vi "read_params.vi"(8 "error in (no error)":errorcluster, 11 "OrthogonalMatchingPursuit in":refnum<class "OrthogonalMatchingPursuit.lvclass">) -> (0 "error out":errorcluster, 2 "params":T1={"n_nonzero_coefs"={"n_nonzero_coefs_type"="None", "n_nonzero_coefs_int"=0.0}, "tol"={"tol_type"="None", "tol_float"=0.0}, "fit_intercept"=TRUE, "normalize"=TRUE, "precompute"={"precompute_type"="auto", "precompute_bool"=FALSE}}, 3 "OrthogonalMatchingPursuit out":refnum<class "OrthogonalMatchingPursuit.lvclass">)   [LabVIEW 2020, in "OrthogonalMatchingPursuit.lvclass"]
uses:
  OrthogonalMatchingPursuit.lvclass
  Controls/orthogonal_matching_pursuit_params.ctl
  OrthogonalMatchingPursuit.lvclass/OrthogonalMatchingPursuit.ctl
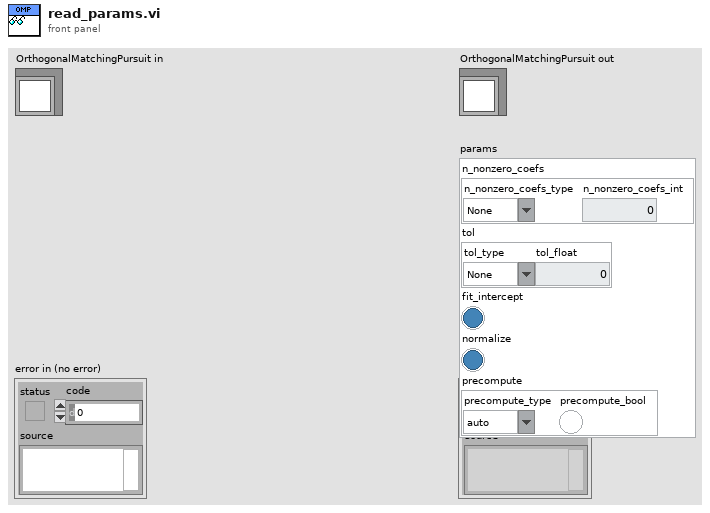
[diagram p1: front panel]
types:
  T1 = typedef "orthogonal_matching_pursuit_params.ctl" = cluster{"n_nonzero_coefs":cluster{"n_nonzero_coefs_type":string, "n_nonzero_coefs_int":dbl}, "tol":cluster{"tol_type":string, "tol_float":dbl}, "fit_intercept":bool, "normalize":bool, "precompute":cluster{"precompute_type":string, "precompute_bool":bool}}
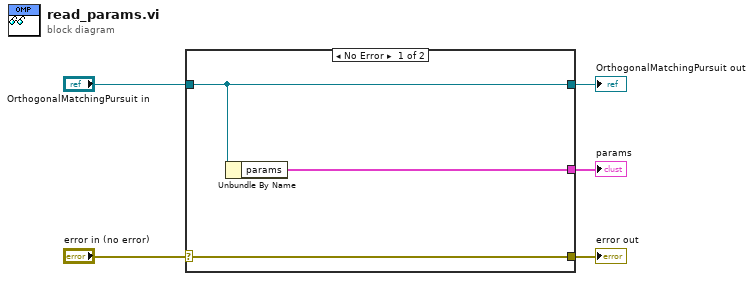
[diagram p0: block diagram]
diagram:
  n1 = case shown="No Error" "error in (no error)" {
    selector: "error in (no error)" -> [w8 w9]
    tunnel: [w8 w9] -> w4
    tunnel: [w7 w10] -> w2
    tunnel: "OrthogonalMatchingPursuit in" -> [w7 w10]
    tunnel: [w6 _] -> w1
    frame No Error {
      n2 = Unbundle By Name(w7) -> ("params"=w6:T1)
    }
    frame Error {
    }
  }
  "error out" <- w4
  "OrthogonalMatchingPursuit out" <- w2
  "params" <- w1
